vi "Check if position is correcct.vi"(8 "error in (no error)":errorcluster, 10 "Tolerance (um)":dbl, 11 "Tomo in":refnum<class "Tomo.lvclass">) -> (0 "error out":errorcluster, 2 "correct?":bool, 3 "Tomo out":refnum<class "Tomo.lvclass">)   [LabVIEW 2012, in "Tomo.lvclass"]
uses:
  Tomo.lvclass
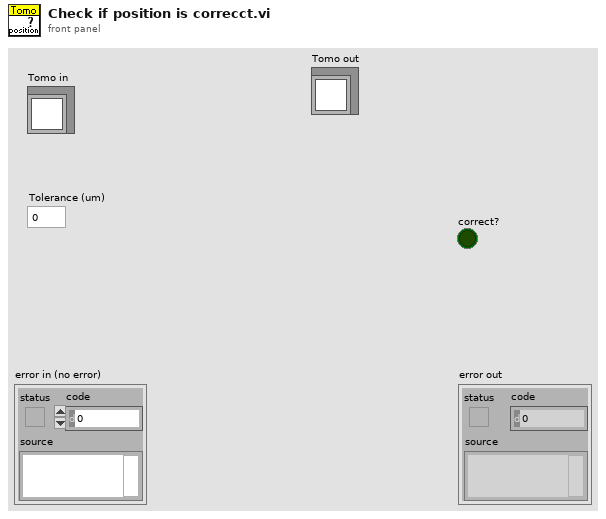
[diagram p1: front panel]
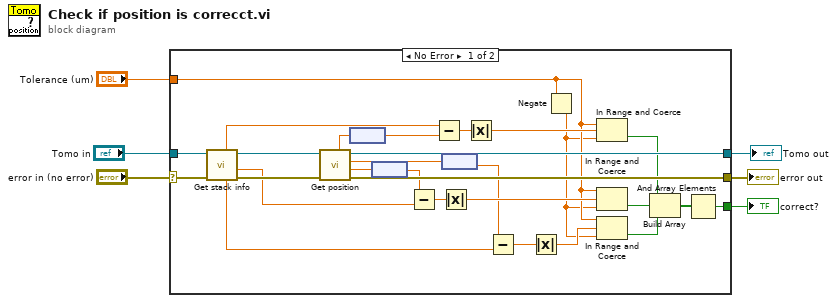
[diagram p0: block diagram]
diagram:
  n1 = case shown="No Error" "error in (no error)" {
    selector: "error in (no error)" -> [w33 w36]
    tunnel: [w31 w36] -> w5
    tunnel: [w29 w35] -> w4
    tunnel: "Tomo in" -> [w34 w35]
    tunnel: "Tolerance (um)" -> [w16 _]
    tunnel: [w10 _] -> w2
    frame No Error {
      n2 = call-dynamic "Get stack info.vi"("error in (no error)"=w33, "Tomo in"=w34) -> ("error out"=w32:errorcluster, "Z start"=w9:dbl, "Tomo out"=w30:refnum<class "Tomo.lvclass">, "Y position"=w8:dbl, "X position"=w7:dbl)  [unwired: 4 in, 1 out]
      n3 = call-dynamic "Get position.vi"("error in (no error)"=w32, "Tomo in"=w30) -> ("error out"=w31:errorcluster, "Z position"=w26:dbl[unit], "Y position"=w24:dbl[unit], "Tomo out"=w29:refnum<class "Tomo.lvclass">, "X position"=w28:dbl[unit])  [unwired: 4 in, 1 out]
      n4 = node(w28) -> (w19:dbl)
      n5 = node(w26) -> (w18:dbl)
      n6 = Subtract(x=w18, y=w9) -> (x-y=w25:dbl)
      n7 = Subtract(x=w7, y=w19) -> (x-y=w27:dbl)
      n8 = Absolute Value(x=w25) -> (abs(x)=w21:dbl)
      n9 = node(w24) -> (w17:dbl)
      n10 = Absolute Value(x=w27) -> (abs(x)=w20:dbl)
      n11 = Subtract(x=w17, y=w8) -> (x-y=w23:dbl)
      n12 = Absolute Value(x=w23) -> (abs(x)=w22:dbl)
      n13 = Negate(x=w16) -> (-x=w15:dbl)
      n14 = In Range and Coerce(upper limit=w16, x=w20, lower limit=w15) -> (In Range?=w14:bool)  [unwired: 1 out]
      n15 = In Range and Coerce(upper limit=w16, x=w21, lower limit=w15) -> (In Range?=w13:bool)  [unwired: 1 out]
      n16 = In Range and Coerce(upper limit=w16, x=w22, lower limit=w15) -> (In Range?=w12:bool)  [unwired: 1 out]
      n17 = Build Array(w14, w13, w12) -> (w11:bool[])
      n18 = And Array Elements(Boolean array=w11) -> (logical AND=w10:bool)
    }
    frame Error {
    }
  }
  "error out" <- w5
  "correct?" <- w2
  "Tomo out" <- w4
